vi "Parse Parameters File.vi"(8 "error in":errorcluster, 11 "path to XML document":path caption="path to parameters xml") -> (0 "error out":errorcluster, 2 "1553 channels":T1[](array[typedef]), 3 "path to XML document out":path caption="path to parameters xml")   [LabVIEW 2020, in "MIL-STD 1553 Import.lvlib"]
uses:
  MIL-STD 1553 Import.lvlib
  Shared/1553 Channel.ctl
  Shared/Address.ctl
  Shared/Message Definition.ctl
  Shared/Message Type.ctl
  Shared/Terminal Endpoint.ctl
  Shared/Parameter Definition.ctl
  3abd4f87-808c-4442-90e1-7f1391a1a862.vi
  3abd4f87-808c-4442-90e1-7f1391a1a862.vi/b1e6fcf8-dac1-42d2-b1fe-151afe06dbd4.vi
  3abd4f87-808c-4442-90e1-7f1391a1a862.vi/b1e6fcf8-dac1-42d2-b1fe-151afe06dbd4.vi/49c1b1ee-2d2a-4a85-8ca5-42123c34e85a.vi
  <vilib>/xml/Load XML File.vi
  Constants.vi
  <vilib>/xml/Get Node Text Content.vi
  <vilib>/Utility/error.llb/Error Cluster From Error Code.vi
  <vilib>/xml/Close Reference(Node).vi
  <resource>/objmgr/DOMUserDefRef.rc
  <vilib>/xml/NI_XML.lvlib
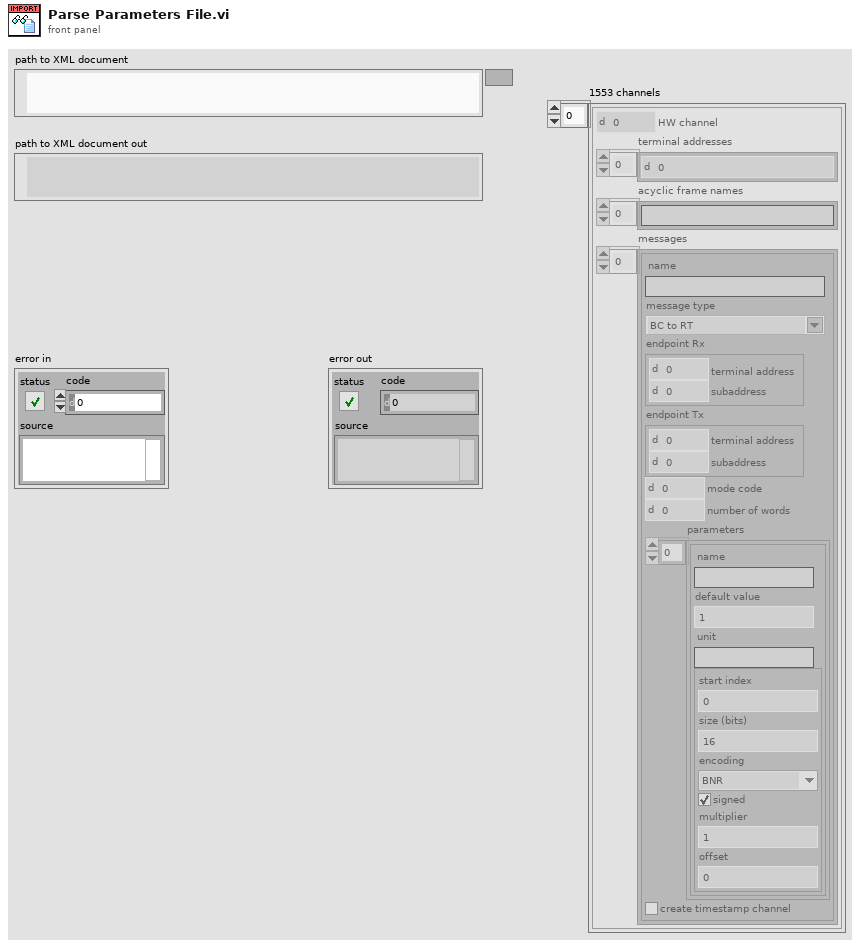
[diagram p1: front panel]
types:
  T1 = typedef "1553 Channel.ctl" = cluster{"HW channel":u16, "terminal addresses":T2[], "acyclic frame names":string[], "messages":T3[]}
  T2 = typedef "Address.ctl" = u16
  T3 = typedef "Message Definition.ctl" = cluster{"name":string, "message type":T4, "endpoint Rx":T5, "endpoint Tx":T5, "mode code":u16, "number of words":u16, "parameters":cluster{"name":string, "default value":dbl, "unit":string, "parameter definition":T6}[], "create timestamp channel":bool}
  T4 = typedef "Message Type.ctl" = string
  T5 = typedef "Terminal Endpoint.ctl" = cluster{"terminal address":T2, "subaddress":T2}
  T6 = typedef "Parameter Definition.ctl" = cluster{"start index":i32, "size (bits)":i32, "encoding":enum16{"BNR", "BCD", "Discrete"}, "signed":bool, "multiplier":dbl, "offset":dbl}
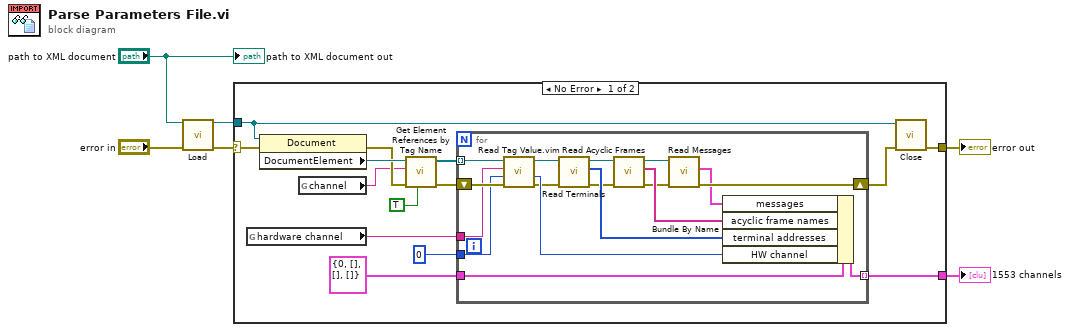
[diagram p0: block diagram]
diagram:
  n1 = call-poly <vilib>:"Load.vi"("path to XML document"="path to XML document", "error in (no error)"="error in") -> ("DOM document out"=w3:refnum<k20>, "error out"=w6:errorcluster)  [unwired: 11 in, 1 out]
  n2 = case shown="No Error" w6 {
    selector: w6 -> [w20 w38]
    tunnel: [w19 w38] -> w4
    tunnel: w3 -> [w18 _]
    tunnel: [w9 _] -> w1
    frame No Error {
      n3 = global read "Constants.vi" "hardware channel"() -> (w11:string)
      n4 = property class="Document"(reference=w18, error in=w20) -> (error out=w16:errorcluster, "DocumentElement"=w17:refnum<k20>)  [unwired: 1 out]
      n5 = global read "Constants.vi" "channel"() -> (w15:string)
      n6 = call "Get Element References by Tag Name.vi"("required (F)"=TRUE, "error in"=w16, "tag name"=w15, "node in"=w17) -> ("error out"=w13:errorcluster, "array of elements"=w14:refnum<k20>[])  [unwired: 6 in]
      n7 = for {
        tunnel: w14 -> [w37] mode=indexing
        shift-right: [w23] -> w8
        shift-left: w13 -> [w36]
        tunnel: T1 {"HW channel"=0, "terminal addresses"=[], "acyclic frame names"=[], "messages"=[]} ("1553 channel") -> [w33]
        tunnel: w11 -> [w35]
        tunnel: u16 0 -> [w34]
        tunnel: [w31] -> w9 mode=indexing
        n8 = call "Read Tag Value.vim"("error in"=w36, "default"=w34, "tag name"=w35, "node in"=w37) -> ("error out"=w30:errorcluster, "value"=w32:u16, "node out"=w29:refnum<k20>)  [unwired: 5 in]
        n9 = call "Read Terminals.vi"("error in"=w30, "channel ref in"=w29) -> ("error out"=w26:errorcluster, "terminal addresses"=w28:T2[], "channel ref out"=w27:refnum<k20>)  [unwired: 7 in]
        n10 = call "Read Acyclic Frames.vi"("error in"=w26, "channel ref in"=w27) -> ("error out"=w24:errorcluster, "acyclic frame names"=w25:string[], "channel ref out"=w22:refnum<k20>)  [unwired: 7 in]
        n11 = call "Read Messages.vi"("error in"=w24, "channel ref in"=w22) -> ("error out"=w23:errorcluster, "messages"=w21:T3[])  [unwired: 7 in, 1 out]
        n12 = Bundle By Name(cluster=w33, "messages"=w21, "acyclic frame names"=w25, "terminal addresses"=w28, "HW channel"=w32) -> (w31:T1)
      }
      n13 = call-poly <vilib>:"Close.vi"("error in (no error)"=w8, "node"=w18) -> ("error out"=w19:errorcluster)  [unwired: 7 in]
    }
    frame Error {
    }
  }
  "error out" <- w4
  "1553 channels" <- w1
  "path to XML document out" <- "path to XML document"
